vi "SmoothPath.vi"(0 "ignoreBall?":bool, 4 "ball":T1, 5 "defesa":bool=TRUE, 6 "Initial State":dbl[](array[numeric]), 7 "Robot in":T2={"id"=0, "function"=enum."Attacker", "x"=0.0, "y"=0.0, "orientation"=0.0, "v_tangent"=0.0, "v_normal"=0.0, "v_ang"=0.0, "kick_x"=0.0, "kick_z"=0.0, "dribble"=FALSE, "Timestamp"=timestamp(0 s since 1904-01-01), "estimatives"={"est_v_tangent"=0.0, "est_v_normal"=0.0, "est_vx"=0.0, "est_vy"=0.0, "Pos Robot Est"=[]}, "dest_x_kick"=0.0, "dest_y_kick"=0.0, "Gap Coord"=[], "States"=enum."GoToTangent", "Path "=[], "Path  Smooth"=[], "Dest"=[], "vx_desired"=0.0, "vy_desired"=0.0, "slowBehavior"=FALSE, "VSSStates"=enum."Pass"}, 8 "our_robots":T2[](array[typedef]), 9 "enemy_robots":T2[](array[typedef]), 10 "Path":dbl[][](array[numeric]), 11 "Goal":dbl[](array[numeric])) -> (2 "SmoothPath":dbl[][](array[numeric]))   [LabVIEW 2023]
uses:
  Vision_class/Old vision/Controls/AI Robot.ctl
  Vision_class/Old vision/Controls/Functions Enum.ctl
  Vision_class/Old vision/Controls/AttackerStates.ctl
  Vision_class/Old vision/Controls/PathDests.ctl
  Vision_class/Old vision/Controls/PathDest.ctl
  Navigation/VSSNavigation/VSSAttackerStates.ctl
  Vision_class/Old vision/SSL Detection Frame Simple Estimator Cameras VelCmd Folder/Core/AI Ball.ctl
panel:
  out "appended array":dbl[][](array[numeric])
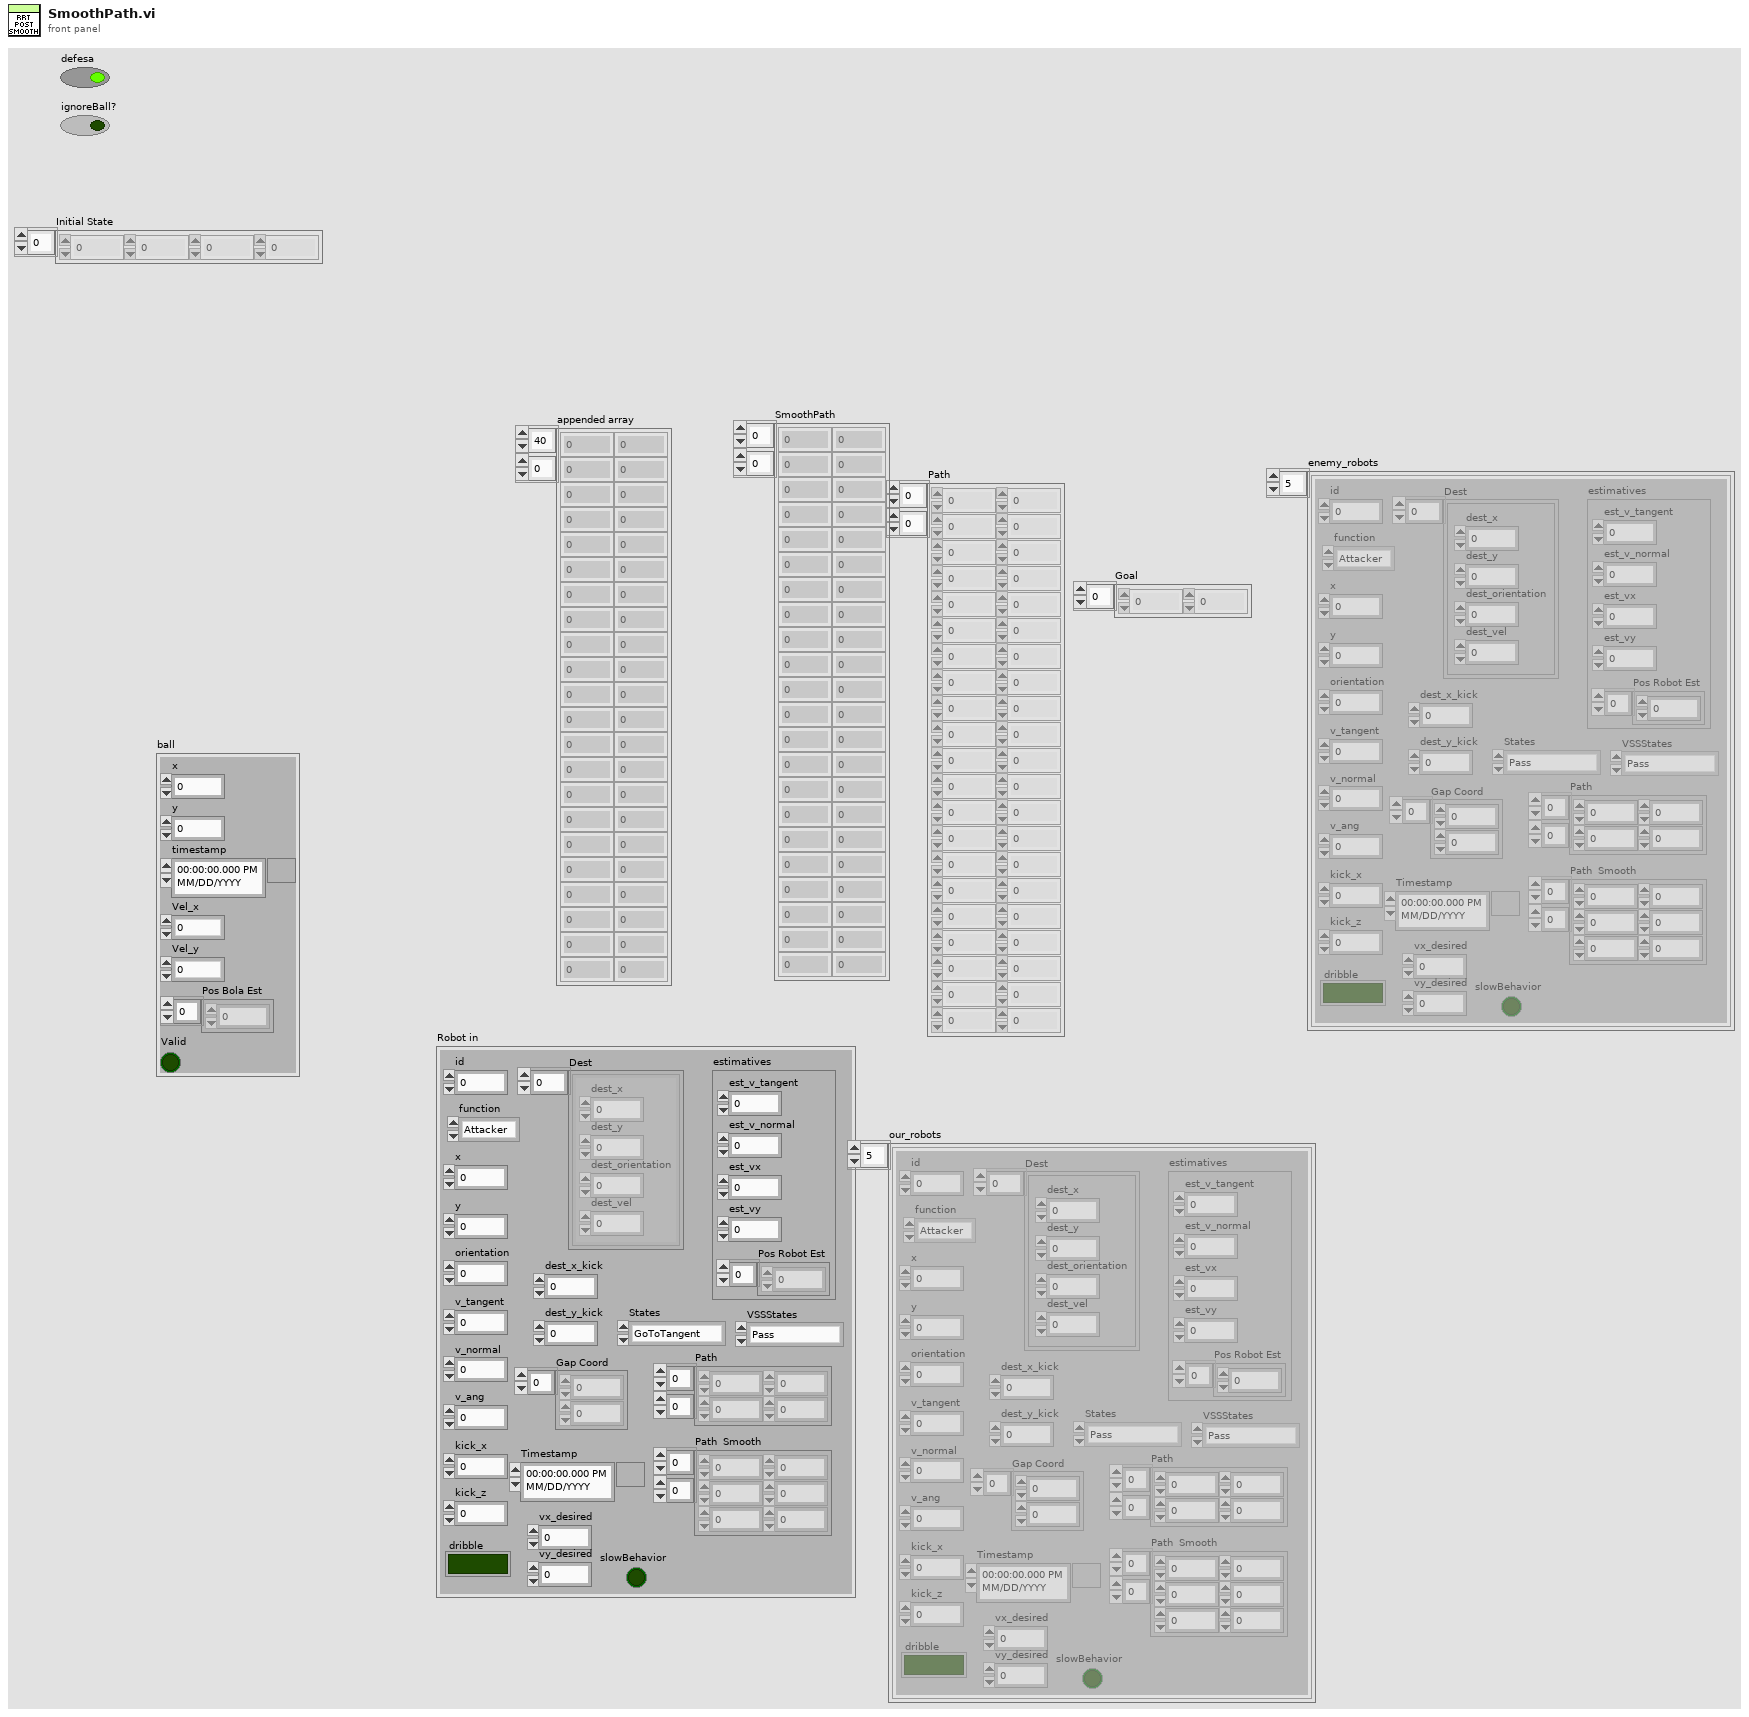
[diagram p1: front panel]
types:
  T1 = typedef "AI Ball.ctl" = cluster{"x":dbl, "y":dbl, "timestamp":timestamp, "Vel_x":dbl, "Vel_y":dbl, "Pos Bola Est":dbl[], "Valid":bool}
  T2 = typedef "AI Robot.ctl" = cluster{"id":u32, "function":T3, "x":dbl, "y":dbl, "orientation":dbl, "v_tangent":dbl, "v_normal":dbl, "v_ang":dbl, "kick_x":dbl, "kick_z":dbl, "dribble":bool, "Timestamp":timestamp, "estimatives":cluster{"est_v_tangent":dbl, "est_v_normal":dbl, "est_vx":dbl, "est_vy":dbl, "Pos Robot Est":dbl[]}, "dest_x_kick":dbl, "dest_y_kick":dbl, "Gap Coord":dbl[], "States":T4, "Path ":dbl[][], "Path  Smooth":dbl[][], "Dest":T5, "vx_desired":dbl, "vy_desired":dbl, "slowBehavior":bool, "VSSStates":T7}
  T3 = typedef "Functions Enum.ctl" = enum16{"2nd Striker", "Attacker", "Goalie", "Defender", "Striker", "Goto 0", "Dummy", "Kicker", "ZigZag 0", "ZigZag 1", "ZigZag 2", "ZigZag 3", "ZigZag 4", "ZigZag 5", "ZigZag 6", "ZigZag 7", "ZigZag 8", ""}
  T4 = typedef "AttackerStates.ctl" = enum16{"Pass", "GoToTangent", "BallGetting", "GoToKick", ""}
  T5 = typedef "PathDests.ctl" = T6[]
  T6 = typedef "PathDest.ctl" = cluster{"dest_x":dbl, "dest_y":dbl, "dest_orientation":dbl, "dest_vel":dbl}
  T7 = typedef "VSSAttackerStates.ctl" = enum16{"Pass", "GoToTangent", "BallGetting", "GoToKick", "Rotate anti-clockwise", "Rotate Clockwise", ""}
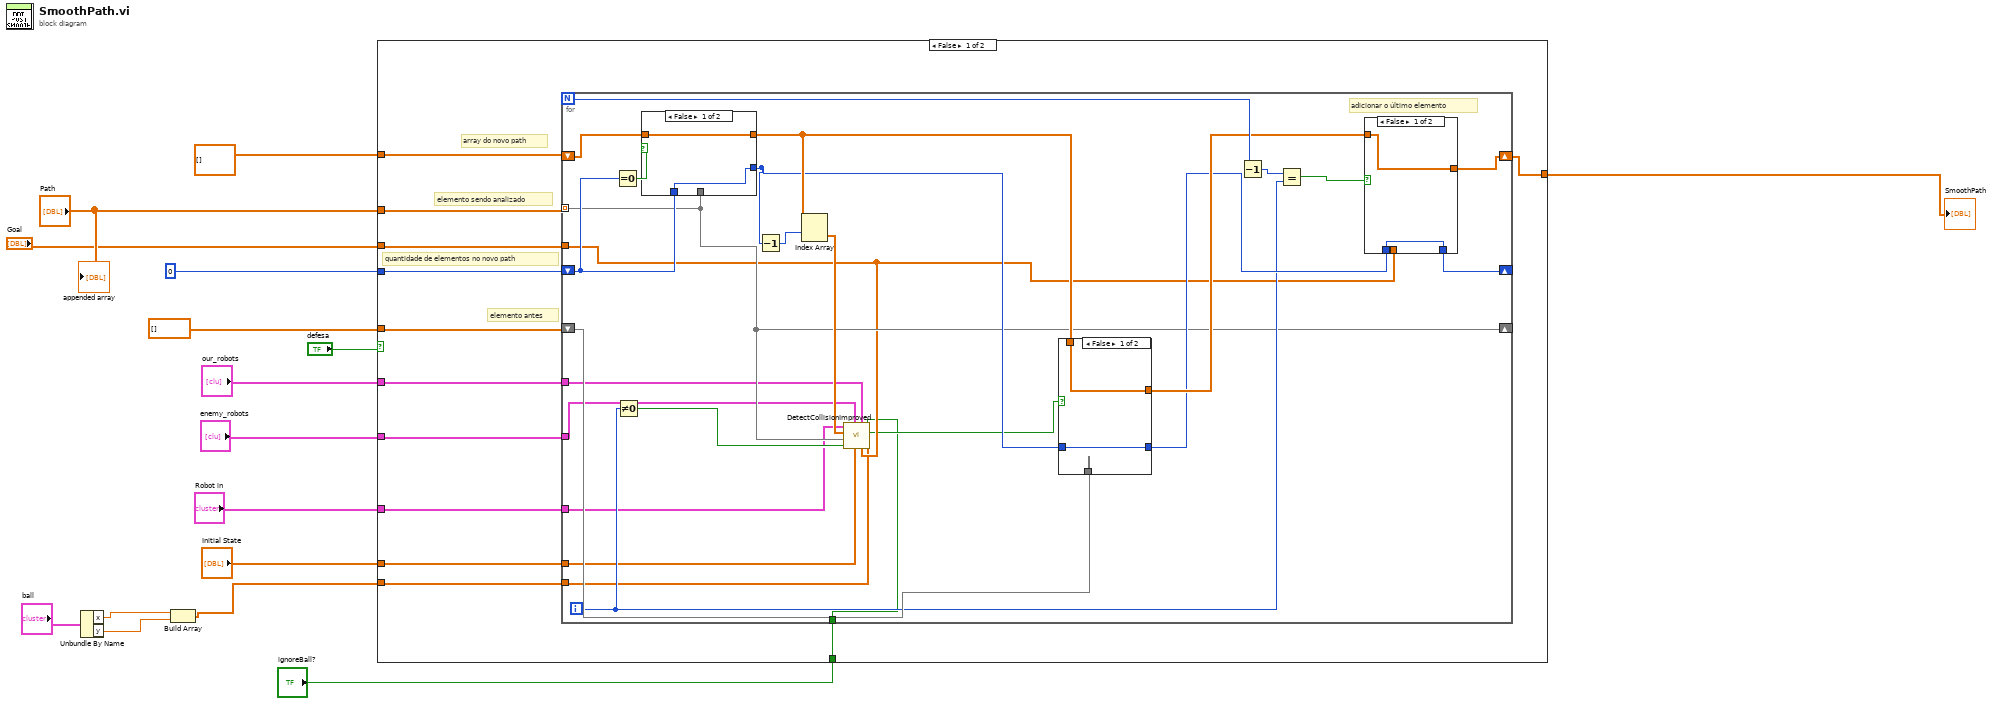
[diagram p0: block diagram]
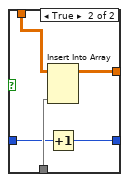
[diagram p2: hidden frame]
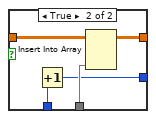
[diagram p3: hidden frame]
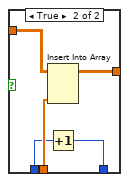
[diagram p4: hidden frame]
diagram:
  n1 = Unbundle By Name("ball") -> ("x"=w4:dbl, "y"=w3:dbl)
  n2 = Build Array(w4, w3) -> (w6:dbl[])
  n3 = case shown="False" "defesa" {
    tunnel: "enemy_robots" -> [w28 _]
    tunnel: dbl[][] [] ("Path") -> [w27 _]
    tunnel: dbl[] [] ("Path") -> [w26 _]
    tunnel: 0 -> [w25 _]
    tunnel: "Robot in" -> [w24 _]
    tunnel: "Path" -> [w23 w76]
    tunnel: "Goal" -> [w22 _]
    tunnel: "Initial State" -> [w21 _]
    tunnel: "our_robots" -> [w20 _]
    tunnel: [w19 w76] -> w7
    tunnel: w6 -> [w18 _]
    tunnel: "ignoreBall?" -> [w17 _]
    frame False {
      # "elemento sendo analizado"
      # "quantidade de elementos no novo path"
      # "elemento antes"
      # "array do novo path"
      n4 = for {
        N -> [w52]
        tunnel: w23 -> [w36] mode=indexing
        tunnel: w28 -> [w34]
        shift-right: [w46] -> w19
        shift-left: w27 -> [w50]
        shift-right: [w36] -> _
        shift-left: w26 -> [w40]
        shift-right: [w45] -> _
        shift-left: w25 -> [w49]
        tunnel: w24 -> [w35]
        tunnel: w22 -> [w33]
        tunnel: w21 -> [w37]
        tunnel: w20 -> [w31]
        tunnel: w18 -> [w30]
        tunnel: w17 -> [w29]
        i -> [w38]
        # "adicionar o último elemento"
        n5 = Equal To 0?(x=w49) -> (x = 0?=w51:bool)
        n6 = Not Equal To 0?(x=w38) -> (x != 0?=w39:bool)
        n7 = case shown="False" w51 {
          tunnel: w36 -> [_ w68]
          tunnel: w50 -> [w62 w67]
          tunnel: [w62 w66] -> w44
          tunnel: w49 -> [w63 w65]
          tunnel: [w63 w64] -> w42
          frame False {
          }
          frame True {
            n8 = Increment(x=w65) -> (x+1=w64:i32)
            n9 = Insert Into Array(array=w67, new element=w68) -> (w66:dbl[][])  [unwired: 2 in]
          }
        }
        n10 = Decrement(x=w42) -> (x-1=w48:i32)
        n11 = Index Array(array=w44, index (row)=w48) -> (element=w47:dbl[])  [unwired: 1 in]
        n12 = call "DetectCollisionImproved.vi"("ball"=w30, "ignoreBall?"=w29, "Goal"=w33, "our_robots"=w31, "Initial State"=w37, "enemy_robots"=w34, "Is not first robot?"=w39, "element being analyzed"=w36, "element already in path"=w47, "Robot in"=w35) -> ("Is there colision?"=w32:bool)  [unwired: 1 in]
        n13 = case shown="False" w32 {
          tunnel: w40 -> [_ w61]
          tunnel: [w55 w60] -> w43
          tunnel: w44 -> [w55 w59]
          tunnel: w42 -> [w56 w58]
          tunnel: [w56 w57] -> w41
          frame False {
          }
          frame True {
            n14 = Insert Into Array(array=w59, new element=w61) -> (w60:dbl[][])  [unwired: 2 in]
            n15 = Increment(x=w58) -> (x+1=w57:i32)
          }
        }
        n16 = Decrement(x=w52) -> (x-1=w53:i32)
        n17 = Equal?(x=w53, y=w38) -> (x = y?=w54:bool)
        n18 = case shown="False" w54 {
          tunnel: w33 -> [_ w75]
          tunnel: w43 -> [w70 w74]
          tunnel: [w70 w73] -> w46
          tunnel: w41 -> [w69 w72]
          tunnel: [w69 w71] -> w45
          frame False {
          }
          frame True {
            n19 = Insert Into Array(array=w74, new element=w75) -> (w73:dbl[][])  [unwired: 2 in]
            n20 = Increment(x=w72) -> (x+1=w71:i32)
          }
        }
      }
    }
    frame True {
    }
  }
  "SmoothPath" <- w7
  "appended array" <- "Path"
